vi "ChangeTileColorShift.vi"(8 "error in (no error)":errorcluster, 10 "Reset":bool, 11 "Engine in":refnum<class "Engine.lvclass">) -> (0 "error out":errorcluster, 3 "Engine out":refnum<class "Engine.lvclass">)   [LabVIEW 2019, in "RT_Game.lvlib" / "Engine.lvclass"]
uses:
  Engine.lvclass
  Engine.lvclass/Engine.ctl
  <vilib>/Utility/error.llb/Error Cluster From Error Code.vi
  <vilib>/rvi/errors/niLvFpgaAdjustHostInterfaceError.vi
  <vilib>/rvi/interface/nirviReadWriteControl/nirviReadWriteControl.xnode
  FPGA_Interface.ctl
  FPGA Bitfiles/myriogameconsole_FPGATarget_Main_ntsPRcBZGxk.lvbitx
  NiFpgaLv.dll
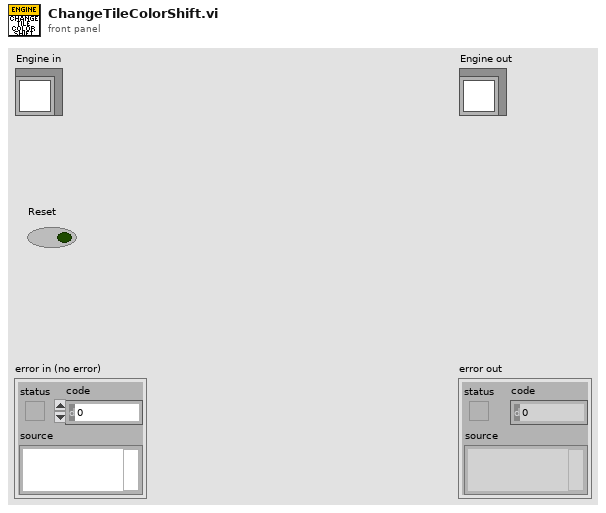
[diagram p1: front panel]
types:
  T1 = typedef "FPGA_Interface.ctl" = refnum<k20>
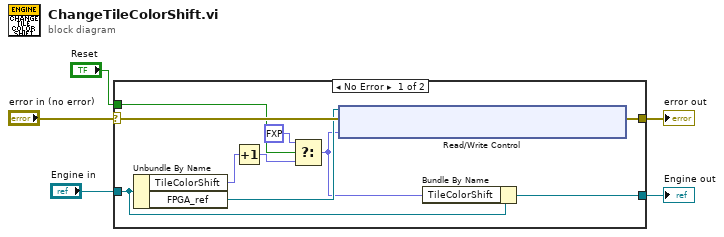
[diagram p0: block diagram]
diagram:
  n1 = case shown="No Error" "error in (no error)" {
    selector: "error in (no error)" -> [w15 w17]
    tunnel: [w14 w17] -> w4
    tunnel: [w11 w16] -> w2
    tunnel: "Engine in" -> [w13 w16]
    tunnel: "Reset" -> [w8 _]
    frame No Error {
      n2 = Unbundle By Name(w13) -> ("TileColorShift"=w10:fxp<+,3,3>, "FPGA_ref"=w12:T1)
      n3 = Increment(x=w10) -> (x+1=w9:fxp<+,3,3>)
      n4 = Select(t=fxp<+,3,3> 0.0, s=w8, f=w9) -> (s? t:f=w6:fxp<+,3,3>)
      n5 = xnode "Read/Write Control"("FPGA VI Reference In"=w12, "error in"=w15, "TileColorShift"=w6) -> ("error out"=w14:errorcluster)  [unwired: 1 out]
      n6 = Bundle By Name(cluster=w13, "TileColorShift"=w6) -> (w11:refnum<class "Engine.lvclass">)
    }
    frame Error {
    }
  }
  "error out" <- w4
  "Engine out" <- w2
